vi "A3200_4_Axis_MoveInc.vi"() -> ()   [LabVIEW 2016]
uses:
  <userlib>/Aerotech A3200/Utility/AxisControl.ctl
  <userlib>/Aerotech A3200/Motion/AbortSingle.vi
  <userlib>/Aerotech A3200/Motion/MoveIncSingle.vi
  <userlib>/Aerotech A3200/Motion/FreerunSingle.vi
  <userlib>/Aerotech A3200/Motion/EnableSingle.vi
  <userlib>/Aerotech A3200/Motion/DisableSingle.vi
  <userlib>/Aerotech A3200/Motion/HomeSingle.vi
  <userlib>/Aerotech A3200/Motion/FaultAckSingle.vi
  <userlib>/Aerotech A3200/Parameters/GetAxisParameterString.vi
  <userlib>/Aerotech A3200/Parameters/GetAxisParameterDouble.vi
  <userlib>/Aerotech A3200/Aerotech VIs.lvlib
panel:
  out "error out":errorcluster
  in  "Reset Controller":bool
  in  "Axes":T1[](array[typedef])
  in  "TaskId":i32(ring)=1 items=["TLibrary", "T01", "T02", "T03", "T04", "T05", "T06", "T07", "T08", "T09", "T10", "T11", "T12", "T13", "T14", "T15", "T16", "T17", "T18", "T19", "T20", "T21", "T22", "T23", "T24", "T25", "T26", "T27", "T28", "T29", "T30", "T31"]
  out "do stop":bool
  in  "Abort":bool
  in  "Disconnect?":bool
  in  "stop":bool
  in  "Status":string
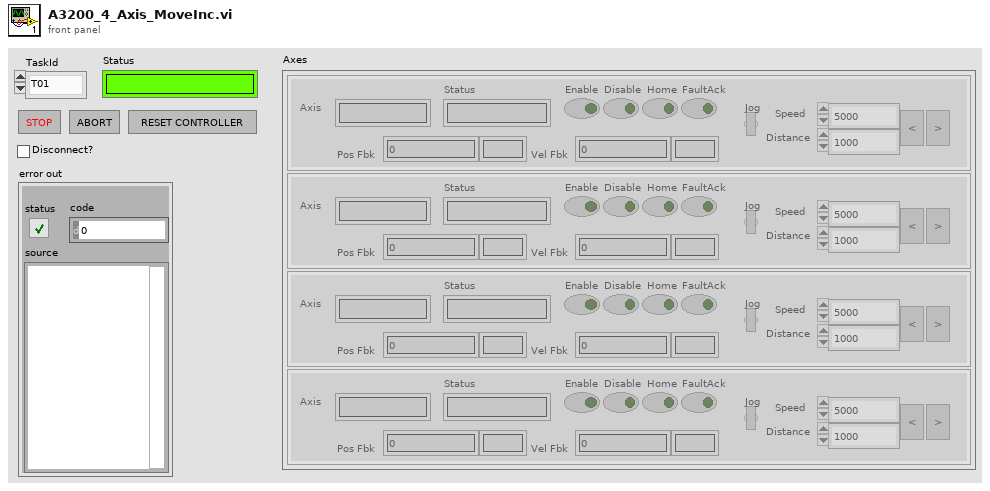
[diagram p1: front panel]
types:
  T1 = typedef "Aerotech VIs.lvlib/AxisControl.ctl" = cluster{"Axis":string, "Enable":bool, "Disable":bool, "Home":bool, "FaultAck":bool, "Jog":bool, "Speed":dbl, "Distance":dbl, "Jog Left":bool, "Jog Right":bool, "Status":string, "Pos Fbk":dbl, "Vel Fbk":dbl, "Pos Units":string, "Vel Units":string}
  T2 = cluster{"new reference":refnum<k24>, "Event Callback":refnum<k27>, "ControllerDiagPacket":refnum<user-event>, "Event Registration Refnum":refnum<event-registration>}
  T3 = typedef "AxisDiagPacket.ctl" = cluster{"Axis Name":string, "Analog Input 0":dbl, "Analog Input 1":dbl, "Axis Fault (num)":i32, "Axis Fault (str)":string, "Axis Fault (bits)":cluster{"AmplifierFault":bool, "AmplifierTemperatureFault":bool, "CcwEndOfTravelLimitFault":bool, "CcwSoftwareLimitFault":bool, "CommunicationLostFault":bool, "CwEndOfTravelLimitFault":bool, "CwSoftwareLimitFault":bool, "EmergencyStopFault":bool, "EncoderFault":bool, "ExternalFault":bool, "FeedbackScalingFault":bool, "GantryMisalignFault ":bool, "HallSensorFault":bool, "InPositionTimeoutFault":bool, "MarkerSearchFault":bool, "MaxVelocityCommandFault":bool, "MotorTemperatureFault":bool, "None":bool, "OverCurrentFault":bool, "PositionErrorFault":bool, "PositionFeedbackFault":bool, "ProbeInputFault":bool, "SafeZoneFault":bool, "VelocityErrorFault":bool, "VelocityFeedbackFault":bool, "VoltageClampFault":bool, "PowerSupplyFault":bool}, "Axis Status (num)":i32, "Axis Status (str)":string, "Axis Status (bits)":cluster{"BacklashActive":bool, "CalibrationEnabled1D":bool, "CalibrationEnabled2D":bool, "CommandValid":bool, "DriveAbortPending":bool, "DrivePending":bool, "Enabling":bool, "GainMappingEnabled":bool, "GantryAligned":bool, "GantryRealigning":bool, "Homed":bool, "Homing":bool, "IFOVEnabled":bool, "Jogging":bool, "JogGenerating":bool, "JoystickControl":bool, "MasterSlaveControl":bool, "MotionBlocked":bool, "MotionClamped":bool, "MoveDone":bool, "None":bool, "NotVirtual":bool, "Profiling":bool, "Stability0":bool, "Stability1":bool, "TrajectoryFiltering":bool, "WaitDone":bool}, "Current Command":sgl, "Current Error":sgl, "Current Feedback":sgl, "Digital Inputs":i32, "Digital Outputs":i32, "Drive Status":i32, "Drive Status (str)":string, "Drive Status (bits)":cluster{"AccelerationPhase":bool, "AutofocusActive":bool, "BrakeOutput":bool, "CcwEndOfTravelLimitInput":bool, "CosineEncoderError":bool, "CurrentClamp":bool, "CwEndOfTravelLimitInput":bool, "DecelerationPhase":bool, "DualLoopActive":bool, "EmergencyStopInput":bool, "Enabled":bool, "EncoderClipping":bool, "GalvoCalibrationEnabled":bool, "GalvoPowerCorrection":bool, "HallAInput":bool, "HallBInput":bool, "HallCInput":bool, "HighResolutionMode":bool, "HomeLimitInput":bool, "InPosition":bool, "InPosition2":bool, "MarkerInput":bool, "MarkerLatch":bool, "MoveActive":bool, "NoMotorSupply":bool, "None":bool, "PowerLimiting":bool, "ProgrammingFlash":bool, "ProgrammingMXH":bool, "PSOHaltLatch":bool, "ServoControl":bool, "SineEncoderError":bool}, "Position Feedback Auxiliary":dbl, "Position Command":dbl, "Position Error":dbl, "Position Feedback":dbl, "Program Position Command":dbl, "Program Position Error":dbl, "Program Position Feedback":dbl, "Velocity Command":dbl, "Velocity Error":dbl, "Velocity Feedback":dbl}
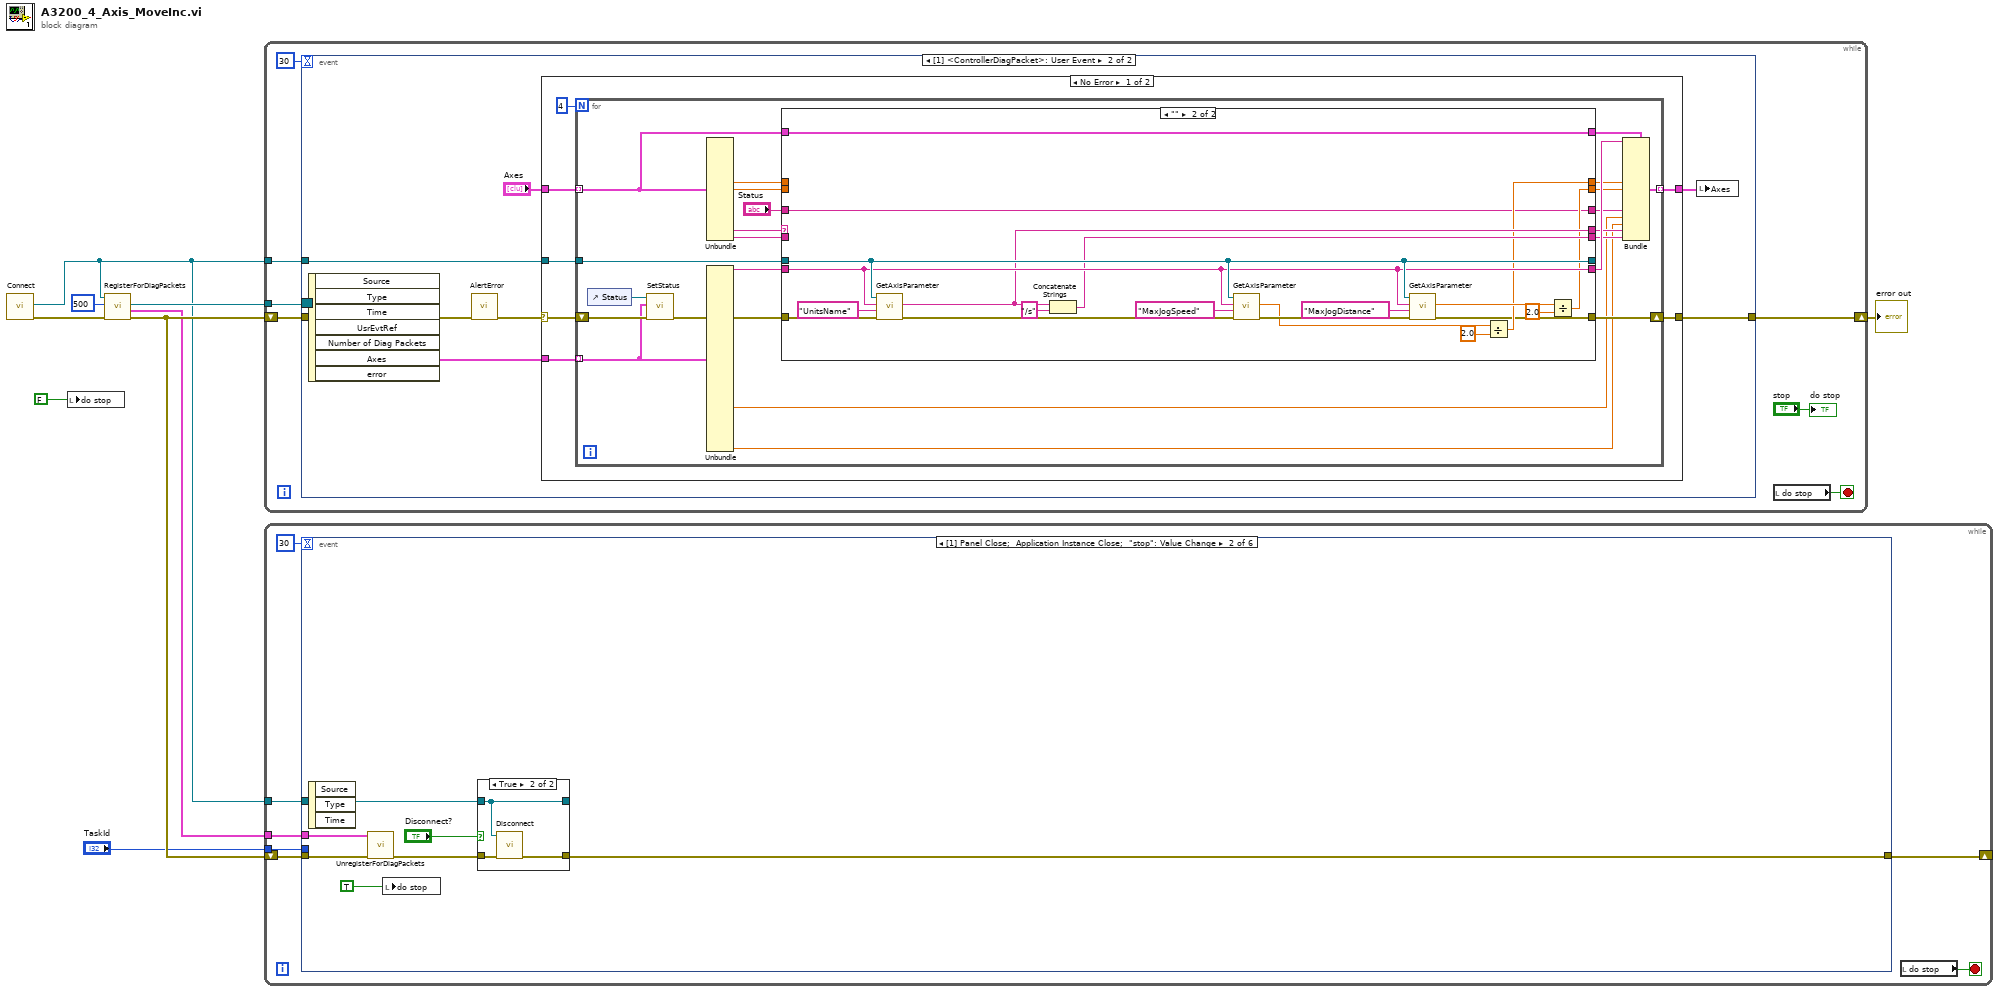
[diagram p0: block diagram]
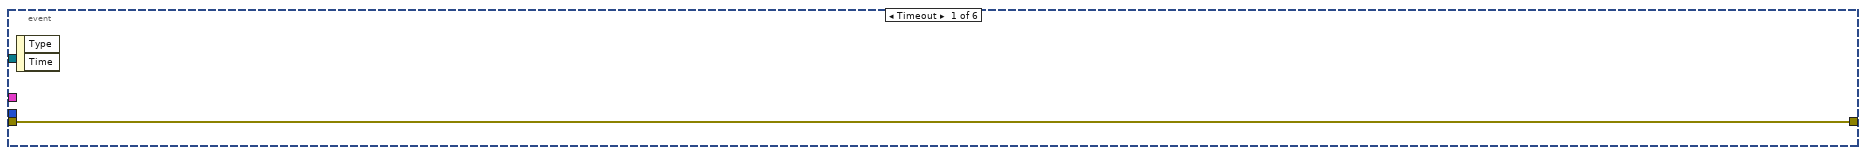
[diagram p2: hidden frame]
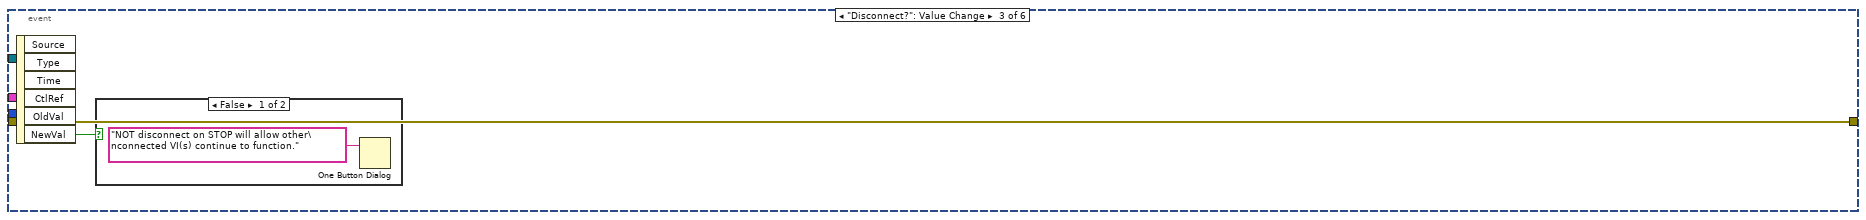
[diagram p4: hidden frame]
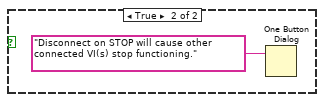
[diagram p5: hidden frame]
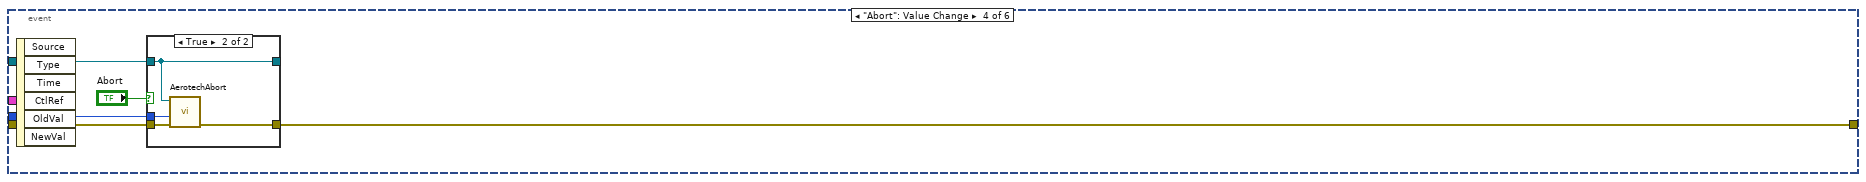
[diagram p6: hidden frame]
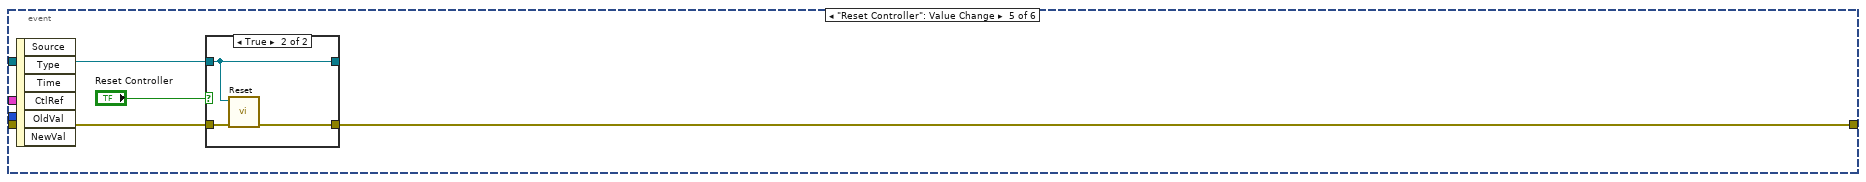
[diagram p8: hidden frame]
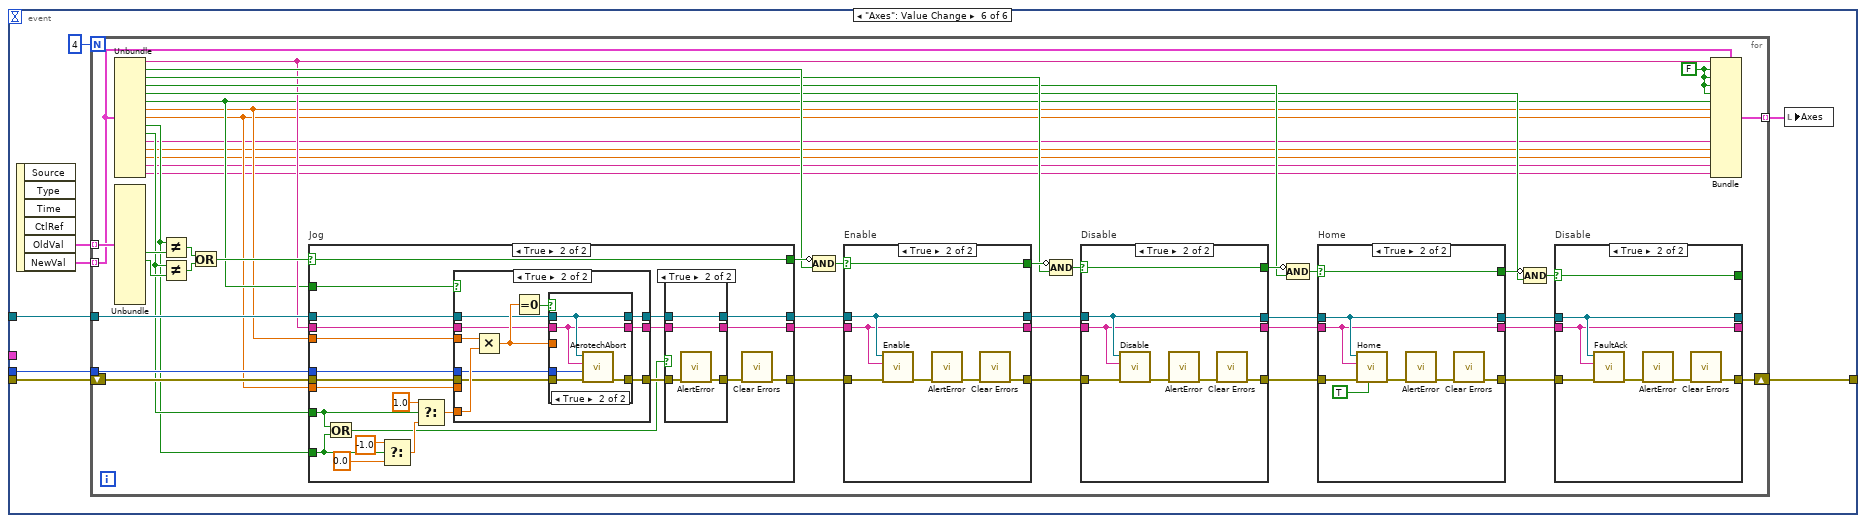
[diagram p10: hidden frame]
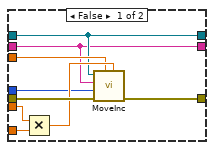
[diagram p17: hidden frame]
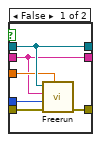
[diagram p18: hidden frame]
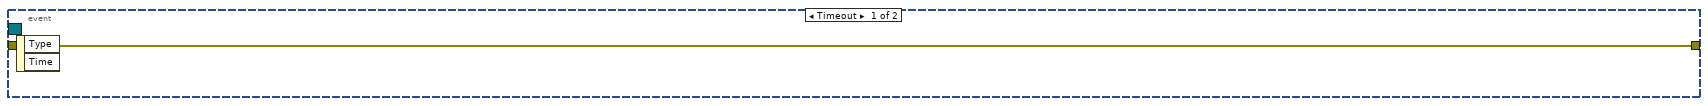
[diagram p19: hidden frame]
diagram:
  n1 = call <userlib>:"Connect.vi"() -> ("error out"=w8:errorcluster, "controller"=w3:refnum<k24>)  [unwired: 10 in]
  n2 = local write "do stop"(FALSE ("do stop")) -> ()
  n3 = call <userlib>:"RegisterForDiagPackets.vi"("error in (no error)"=w8, "refresh interval (default)"=500, "Controller in"=w3) -> ("error out"=w7:errorcluster, "Event Metadata"=w5:T2, "Event Registration Refnum"=w9:refnum<event-registration>)  [unwired: 4 in, 1 out]
  n4 = while {
    tunnel: w9 -> [w13]
    tunnel: w3 -> [w16]
    shift-right: [w14] -> w1
    shift-left: w7 -> [w15]
    stop <- w11 stop-if-true
    n5 = event shown="[1] <ControllerDiagPacket>: User Event" {
      selector: w13 -> [_ _]
      dyn-events: _ -> [_ _]
      timeout: 30 -> [_ _]
      tunnel: w16 -> [_ w24]
      tunnel: w15 -> [w17 w22]
      tunnel: [w17 w23] -> w14
      event Timeout {
        n6 = event-data() -> ()  [unwired: 1 in, 2 out]
      }
      event User Event {
        n7 = event-data() -> ("Axes"=w18:T3[])  [unwired: 1 in, 6 out]
        n8 = call <userlib>:"AlertError.vi"("error in (no error)"=w22) -> ("error out"=w21:errorcluster)  [unwired: 10 in]
        n9 = case shown="No Error" w21 {
          selector: w21 -> [w29 w85]
          tunnel: w24 -> [w31 _]
          tunnel: [w30 w85] -> w23
          tunnel: "Axes" -> [w28 w84]
          tunnel: [w26 w84] -> w19
          tunnel: w18 -> [w25 _]
          frame No Error {
            n10 = for {
              N: 4 -> [_]
              tunnel: w31 -> [w52]
              shift-right: [w51] -> w30
              shift-left: w29 -> [w50]
              tunnel: w28 -> [w48] mode=indexing
              tunnel: [w33] -> w26 mode=indexing
              tunnel: w25 -> [w32] mode=indexing
              n11 = control-ref of="Status"() -> (w53:refnum<vi>)
              n12 = call <userlib>:"SetStatus.vi"("error in (no error)"=w50, "AxisDiagPacket"=w32, "Status string"=w53) -> ("error out"=w49:errorcluster)  [unwired: 8 in]
              n13 = Unbundle(w48) -> ("Speed"=w39:dbl, "Distance"=w38:dbl, "Pos Units"=w44:string, "Vel Units"=w42:string)  [unwired: 11 out]
              n14 = Unbundle(w32) -> ("Axis Name"=w54:string, "Position Feedback"=w37:dbl, "Velocity Feedback"=w36:dbl)  [unwired: 24 out]
              n15 = case shown="\"\"" w44 {
                selector: w44 -> [w59 _]
                tunnel: w54 -> [w61 w73]
                tunnel: w52 -> [w62 w74]
                tunnel: w49 -> [w63 w82]
                tunnel: [w63 w65] -> w51
                tunnel: [w62 w74] -> _
                tunnel: [w61 w73] -> w46
                tunnel: w48 -> [w60 w70]
                tunnel: [w60 w70] -> w47
                tunnel: [w59 w69] -> w45
                tunnel: [w58 w68] -> w43
                tunnel: w42 -> [w58 _]
                tunnel: [w57 w67] -> w41
                tunnel: [w56 w66] -> w40
                tunnel: w39 -> [w57 _]
                tunnel: w38 -> [w56 _]
                tunnel: [w55 w64] -> w35
                tunnel: "Status" -> [w55 w64]
                frame Default {
                }
                frame "" {
                  n16 = call-poly <userlib>:"GetAxisParameter.vi"("error in (no error)"=w82, "Parameter Name"="UnitsName" ("parameter name"), "axis name"=w73, "controller in"=w74) -> ("error out"=w79:errorcluster, "value"=w69:string)  [unwired: 5 in, 1 out]
                  n17 = Concatenate Strings(w69, "/s" ("string")) -> (w68:string)
                  n18 = call-poly <userlib>:"GetAxisParameter.vi"("error in (no error)"=w79, "Parameter Name"="MaxJogSpeed" ("parameter name"), "axis name"=w73, "controller in"=w74) -> ("error out"=w80:errorcluster, "value"=w76:dbl)  [unwired: 5 in, 1 out]
                  n19 = call-poly <userlib>:"GetAxisParameter.vi"("error in (no error)"=w80, "Parameter Name"="MaxJogDistance" ("parameter name"), "axis name"=w73, "controller in"=w74) -> ("error out"=w65:errorcluster, "value"=w75:dbl)  [unwired: 5 in, 1 out]
                  n20 = Divide(x=w76, y=2.0) -> (x/y=w67:dbl)
                  n21 = Divide(x=w75, y=2.0) -> (x/y=w66:dbl)
                }
              }
              n22 = Bundle(cluster=w47, "Axis"=w46, "Speed"=w41, "Distance"=w40, "Status"=w35, "Pos Fbk"=w37, "Vel Fbk"=w36, "Pos Units"=w45, "Vel Units"=w43) -> (w33:T1)  [unwired: 7 in]
            }
          }
          frame Error {
          }
        }
        n23 = local write "Axes"(w19) -> ()
      }
    }
    n24 = local read "do stop"() -> (w11:bool)
    "do stop" <- "stop"
  }
  "error out" <- w1
  n25 = while {
    tunnel: w3 -> [w89]
    shift-right: [w91] -> _
    shift-left: w7 -> [w92]
    tunnel: w5 -> [w90]
    tunnel: "TaskId" -> [w88]
    stop <- w86 stop-if-true
    n26 = event shown="[1] Panel Close;  Application Instance Close;  \"stop\": Value Change" {
      selector: _ -> [_ _ _ _ _ _]
      dyn-events: _ -> [_ _ _ _ _ _]
      timeout: 30 -> [_ _ _ _ _ _]
      tunnel: w92 -> [w93 w95 w106 w113 w124 w137]
      tunnel: [w93 w100 w106 w112 w121 w134] -> w91
      tunnel: w89 -> [_ w99 _ w110 w123 w135]
      tunnel: w90 -> [_ w94 _ _ _ _]
      tunnel: w88 -> [_ _ _ w111 _ w136]
      event Timeout {
        n27 = event-data() -> ()  [unwired: 1 in, 2 out]
      }
      event Panel Close; Application Instance Close; "stop": Value Change {
        n28 = event-data() -> ()  [unwired: 1 in, 3 out]
        n29 = call <userlib>:"UnregisterForDiagPackets.vi"("Event Metadata"=w94, "error in (no error)"=w95) -> ("error out"=w96:errorcluster)  [unwired: 8 in]
        n30 = local write "do stop"(TRUE) -> ()
        n31 = case shown="True" "Disconnect?" {
          tunnel: w96 -> [w102 w105]
          tunnel: [w102 w104] -> w100
          tunnel: w99 -> [w101 w103]
          tunnel: [w101 w103] -> _
          frame False {
          }
          frame True {
            n32 = call <userlib>:"Disconnect.vi"("error in (no error)"=w105, "controller"=w103) -> ("error out"=w104:errorcluster)  [unwired: 9 in]
          }
        }
      }
      event "Disconnect?": Value Change {
        n33 = event-data() -> ("NewVal"=w107:bool)  [unwired: 1 in, 5 out]
        n34 = case shown="False" w107 {
          frame False {
            n35 = One Button Dialog(message="NOT disconnect on STOP will allow other\nconnected VI(s) continue to function.") -> ()  [unwired: 1 in, 1 out]
          }
          frame True {
            n36 = One Button Dialog(message="Disconnect on STOP will cause other connected VI(s) stop functioning.") -> ()  [unwired: 1 in, 1 out]
          }
        }
      }
      event "Abort": Value Change {
        n37 = event-data() -> ()  [unwired: 1 in, 6 out]
        n38 = case shown="True" "Abort" {
          tunnel: w113 -> [w116 w120]
          tunnel: [w116 w119] -> w112
          tunnel: w111 -> [_ w118]
          tunnel: w110 -> [w115 w117]
          tunnel: [w115 w117] -> _
          frame False {
          }
          frame True {
            n39 = call-poly <userlib>:"AerotechAbort.vi"("error in (no error)"=w120, "taskId"=w118, "controller in"=w117) -> ("error out"=w119:errorcluster)  [unwired: 7 in, 1 out]
          }
        }
      }
      event "Reset Controller": Value Change {
        n40 = event-data() -> ()  [unwired: 1 in, 6 out]
        n41 = case shown="True" "Reset Controller" {
          tunnel: w124 -> [w126 w129]
          tunnel: [w126 w128] -> w121
          tunnel: w123 -> [w125 w127]
          tunnel: [w125 w127] -> _
          frame False {
          }
          frame True {
            n42 = call <userlib>:"Reset.vi"("error in (no error)"=w129, "controller in"=w127) -> ("error out"=w128:errorcluster)  [unwired: 8 in, 1 out]
          }
        }
      }
      event "Axes": Value Change {
        n43 = event-data() -> ("OldVal"=w133:T1[], "NewVal"=w132:T1[])  [unwired: 1 in, 4 out]
        n44 = for {
          N: 4 -> [_]
          tunnel: w136 -> [w184]
          tunnel: w135 -> [w183]
          shift-right: [w154] -> w134
          shift-left: w137 -> [w185]
          tunnel: w133 -> [w182] mode=indexing
          tunnel: w132 -> [w149] mode=indexing
          tunnel: [w138] -> w131 mode=indexing
          w147 = FALSE ("Enable")
          n45 = Unbundle(w149) -> ("Axis"=w148:string, "Enable"=w171:bool, "Disable"=w161:bool, "Home"=w158:bool, "FaultAck"=w150:bool, "Jog"=w146:bool, "Speed"=w145:dbl, "Distance"=w144:dbl, "Jog Left"=w175:bool, "Jog Right"=w176:bool, "Status"=w139:string, "Pos Fbk"=w140:dbl, "Vel Fbk"=w141:dbl, "Pos Units"=w142:string, "Vel Units"=w143:string)
          n46 = Unbundle(w182) -> ("Jog Left"=w179:bool, "Jog Right"=w178:bool)  [unwired: 13 out]
          n47 = Not Equal?(x=w175, y=w179) -> (x != y?=w181:bool)
          n48 = Not Equal?(x=w176, y=w178) -> (x != y?=w180:bool)
          n49 = Or(x=w181, y=w180) -> (x .or. y?=w177:bool)
          n50 = case "Jog" shown="True" w177 {
            selector: w177 -> [w233 w239]
            tunnel: w148 -> [w231 w252]
            tunnel: w185 -> [w234 w251]
            tunnel: w184 -> [_ w247]
            tunnel: w183 -> [w232 w246]
            tunnel: [w234 w245] -> w173
            tunnel: w176 -> [_ w244]
            tunnel: w175 -> [_ w243]
            tunnel: w146 -> [_ w242]
            tunnel: w145 -> [_ w241]
            tunnel: w144 -> [_ w240]
            tunnel: [w233 w239] -> w172
            tunnel: [w232 w236] -> w170
            tunnel: [w231 w235] -> w169
            frame False {
            }
            frame True {
              n51 = Or(x=w244, y=w243) -> (x .or. y?=w248:bool)
              n52 = Select(t=-1.0, s=w243, f=0.0) -> (s? t:f=w257:dbl)
              n53 = Select(t=1.0, s=w244, f=w257) -> (s? t:f=w253:dbl)
              n54 = case shown="True" w242 {
                tunnel: w241 -> [w268 w284]
                tunnel: w240 -> [w273 _]
                tunnel: w253 -> [w272 w283]
                tunnel: w251 -> [w271 w282]
                tunnel: w252 -> [w265 w275]
                tunnel: [w270 w281] -> w249
                tunnel: w247 -> [w267 w280]
                tunnel: w246 -> [w266 w277]
                tunnel: [w266 w276] -> w238
                tunnel: [w265 w274] -> w237
                frame False {
                  n55 = Multiply(x=w273, y=w272) -> (x*y=w269:dbl)
                  n56 = call-poly <userlib>:"MoveInc.vi"("distance"=w269, "speed"=w268, "error in (no error)"=w271, "taskId"=w267, "axis name"=w265, "controller in"=w266) -> ("error out"=w270:errorcluster)  [unwired: 4 in, 1 out]
                }
                frame True {
                  n57 = Multiply(x=w284, y=w283) -> (x*y=w278:dbl)
                  n58 = Equal To 0?(x=w278) -> (x = 0?=w279:bool)
                  n59 = case shown="True" w279 {
                    tunnel: w282 -> [w290 w295]
                    tunnel: [w289 w294] -> w281
                    tunnel: w278 -> [w286 _]
                    tunnel: w280 -> [w288 w293]
                    tunnel: [w287 w292] -> w276
                    tunnel: w277 -> [w287 w292]
                    tunnel: w275 -> [w285 w291]
                    tunnel: [w285 w291] -> w274
                    frame False {
                      n60 = call-poly <userlib>:"Freerun.vi"("speed"=w286, "error in (no error)"=w290, "taskId"=w288, "axis name"=w285, "controller in"=w287) -> ("error out"=w289:errorcluster)  [unwired: 5 in, 1 out]
                    }
                    frame True {
                      n61 = call-poly <userlib>:"AerotechAbort.vi"("error in (no error)"=w295, "taskId"=w293, "axis name? (all)"=w291, "controller in"=w292) -> ("error out"=w294:errorcluster)  [unwired: 6 in, 1 out]
                    }
                  }
                }
              }
              n62 = case shown="True" w248 {
                tunnel: [w260 w264] -> w250
                tunnel: w249 -> [w260 w263]
                tunnel: w238 -> [w259 w261]
                tunnel: w237 -> [w258 w262]
                tunnel: [w258 w262] -> w235
                tunnel: [w259 w261] -> w236
                frame False {
                }
                frame True {
                  n63 = call <userlib>:"AlertError.vi"("error in (no error)"=w263) -> ("error out"=w264:errorcluster)  [unwired: 10 in]
                }
              }
              n64 = call <vilib>:"Clear Errors.vi"("error in (no error)"=w250) -> ("error out"=w245:errorcluster)  [unwired: 5 in, 1 out]
            }
          }
          n65 = Compound Arithmetic op=AND(invert w172, w171) -> (w174:bool)
          n66 = case "Enable" shown="True" w174 {
            selector: w174 -> [w220 w224]
            tunnel: [w223 w228] -> w165
            tunnel: w173 -> [w223 w227]
            tunnel: [w222 w226] -> w164
            tunnel: w170 -> [w222 w226]
            tunnel: [w221 w225] -> w163
            tunnel: w169 -> [w221 w225]
            tunnel: [w220 w224] -> w162
            frame False {
            }
            frame True {
              n67 = call-poly <userlib>:"Enable.vi"("error in (no error)"=w227, "axis name"=w225, "controller in"=w226) -> ("error out"=w230:errorcluster)  [unwired: 7 in, 1 out]
              n68 = call <userlib>:"AlertError.vi"("error in (no error)"=w230) -> ("error out"=w229:errorcluster)  [unwired: 10 in]
              n69 = call <vilib>:"Clear Errors.vi"("error in (no error)"=w229) -> ("error out"=w228:errorcluster)  [unwired: 5 in, 1 out]
            }
          }
          n70 = Compound Arithmetic op=AND(invert w162, w161) -> (w168:bool)
          n71 = case "Disable" shown="True" w168 {
            selector: w168 -> [w186 w190]
            tunnel: [w189 w194] -> w160
            tunnel: w165 -> [w189 w193]
            tunnel: [w188 w192] -> w157
            tunnel: w164 -> [w188 w192]
            tunnel: [w187 w191] -> w156
            tunnel: w163 -> [w187 w191]
            tunnel: [w186 w190] -> w159
            frame False {
            }
            frame True {
              n72 = call-poly <userlib>:"Disable.vi"("error in (no error)"=w193, "axis name"=w191, "controller in"=w192) -> ("error out"=w196:errorcluster)  [unwired: 7 in, 1 out]
              n73 = call <userlib>:"AlertError.vi"("error in (no error)"=w196) -> ("error out"=w195:errorcluster)  [unwired: 10 in]
              n74 = call <vilib>:"Clear Errors.vi"("error in (no error)"=w195) -> ("error out"=w194:errorcluster)  [unwired: 5 in, 1 out]
            }
          }
          n75 = Compound Arithmetic op=AND(invert w159, w158) -> (w167:bool)
          n76 = case "Home" shown="True" w167 {
            selector: w167 -> [w208 w213]
            tunnel: [w211 w217] -> w155
            tunnel: w160 -> [w211 w216]
            tunnel: [w210 w215] -> w153
            tunnel: w157 -> [w210 w215]
            tunnel: [w209 w214] -> w152
            tunnel: w156 -> [w209 w214]
            tunnel: [w208 w213] -> w151
            frame False {
            }
            frame True {
              n77 = call-poly <userlib>:"Home.vi"("return immediately"=TRUE, "error in (no error)"=w216, "axis name"=w214, "controller in"=w215) -> ("error out"=w219:errorcluster)  [unwired: 6 in, 1 out]
              n78 = call <userlib>:"AlertError.vi"("error in (no error)"=w219) -> ("error out"=w218:errorcluster)  [unwired: 10 in]
              n79 = call <vilib>:"Clear Errors.vi"("error in (no error)"=w218) -> ("error out"=w217:errorcluster)  [unwired: 5 in, 1 out]
            }
          }
          n80 = Compound Arithmetic op=AND(invert w151, w150) -> (w166:bool)
          n81 = case "Disable" shown="True" w166 {
            selector: w166 -> [w197 w203]
            tunnel: [w198 w205] -> w154
            tunnel: w155 -> [w198 w204]
            tunnel: [w200 w202] -> _
            tunnel: w153 -> [w200 w202]
            tunnel: [w199 w201] -> _
            tunnel: w152 -> [w199 w201]
            tunnel: [w197 w203] -> _
            frame False {
            }
            frame True {
              n82 = call-poly <userlib>:"FaultAck.vi"("error in (no error)"=w204, "axis name"=w201, "controller in"=w202) -> ("error out"=w207:errorcluster)  [unwired: 7 in, 1 out]
              n83 = call <userlib>:"AlertError.vi"("error in (no error)"=w207) -> ("error out"=w206:errorcluster)  [unwired: 10 in]
              n84 = call <vilib>:"Clear Errors.vi"("error in (no error)"=w206) -> ("error out"=w205:errorcluster)  [unwired: 5 in, 1 out]
            }
          }
          n85 = Bundle(cluster=w149, "Axis"=w148, "Enable"=w147, "Disable"=w147, "Home"=w147, "FaultAck"=w147, "Jog"=w146, "Speed"=w145, "Distance"=w144, "Status"=w139, "Pos Fbk"=w140, "Vel Fbk"=w141, "Pos Units"=w142, "Vel Units"=w143) -> (w138:T1)  [unwired: 2 in]
        }
        n86 = local write "Axes"(w131) -> ()
      }
    }
    n87 = local read "do stop"() -> (w86:bool)
  }
